vi "Firmware Wizard.vi"() -> ()   [LabVIEW 2011, in "LVH-LINX.lvlib"]
doc: "Wizard for uploading firmware to LINX devices."
uses:
  vi.lib/LabVIEW Hacker/LINX/LVH-LINX.lvlib
  vi.lib/LabVIEW Hacker/LINX/Private/Type Defs/Device Family.ctl
  vi.lib/LabVIEW Hacker/LINX/Private/Type Defs/Devices/Device Type.ctl
  vi.lib/LabVIEW Hacker/LINX/Private/Device/Type Defs/Wifi Config.ctl
  vi.lib/LabVIEW Hacker/LINX/Private/Type Defs/WIFI Security Type.ctl
  vi.lib/LabVIEW Hacker/LINX/Private/Type Defs/Deploy Firmware State.ctl
  vi.lib/LabVIEW Hacker/LINX/Private/Type Defs/All Firmware Data FGV States.ctl
  vi.lib/LabVIEW Hacker/LINX/Private/Device/Type Defs/Firmware Interface.ctl
  vi.lib/LabVIEW Hacker/LINX/Private/Device/Type Defs/TCP Config.ctl
  <vilib>/LabVIEW Hacker/LVH-Toolbox/Common/LVH-Common.lvlib
  vi.lib/LabVIEW Hacker/LINX/Private/Device/Device.lvlib
panel:
  out "Error Out":errorcluster
  out "Log Path":path
  in  "Device Family Enum":T1 items=["National Instruments", "Digilent", "Arduino"]
  in  "Error In":errorcluster
  out "Tab Control":T2(tab)=enum."Device"
  in  "Firmware Available?":string
  in  "Settings Button":bool
  out "Device Image":picture
  in  "Device Help":bool
  in  "Device Type":T3 items=["Arduino Leonardo", "Arduino Mega2560", "Arduino Nano", "Arduino Pro Micro", "Arduino Uno"]
  in  "Device Family":T1 items=["Arduino", "Digilent", "PJRC"]
  in  "Device Cancel":bool
  in  "Device Next":bool
  in  "Firmware Program Interface":u16(ring) items=["Serial / USB"]
  in  "Config Message":string
  in  "Int Help":bool
  in  "Int Previous":bool
  in  "Int Cancel":bool
  in  "Int Next":bool
  out "Interface Config":enum32{"N/A", "Serial / USB", "USB", "TCP"}(tab)=enum."Serial / USB"
  in  "Upload COM Port":refnum<visa-resource-name>="ASRL1::INSTR"
  out "Firmware Configuration":enum32{"Serial", "Ethernet", "WIFI"}(tab)=enum."WIFI"
  in  "Port":u16=927
  in  "IP Address":string="192.168.1.27"
  in  "Wifi Configuration":T4
  in  "Firmware Description":string
  in  "FWV Help":bool
  in  "FWV Cancel":bool
  in  "FWV Next":bool
  in  "FWV Previous":bool
  in  "Firmware Version":u16(ring) items=["LINX - Serial / USB", "LINX - Serial / USB (Debug)"]
  out "Deploy Progress Note":string
  in  "Deploy  Progress Bar":u8(slide) scale=0.0..100.0
  in  "View Log":bool
  in  "LINX Forum Link":string="www.labviewhacker.com/forums/linx"
  in  "LINX Landing Page Link":string="www.labviewhacker.com/linx"
  in  "Summary Launch Example":bool
  in  "Summary Text":string
  in  "Summary Next":bool
  in  "Summary Help":bool
  # "Ethernet Settings"
  # "WIFI Settings"
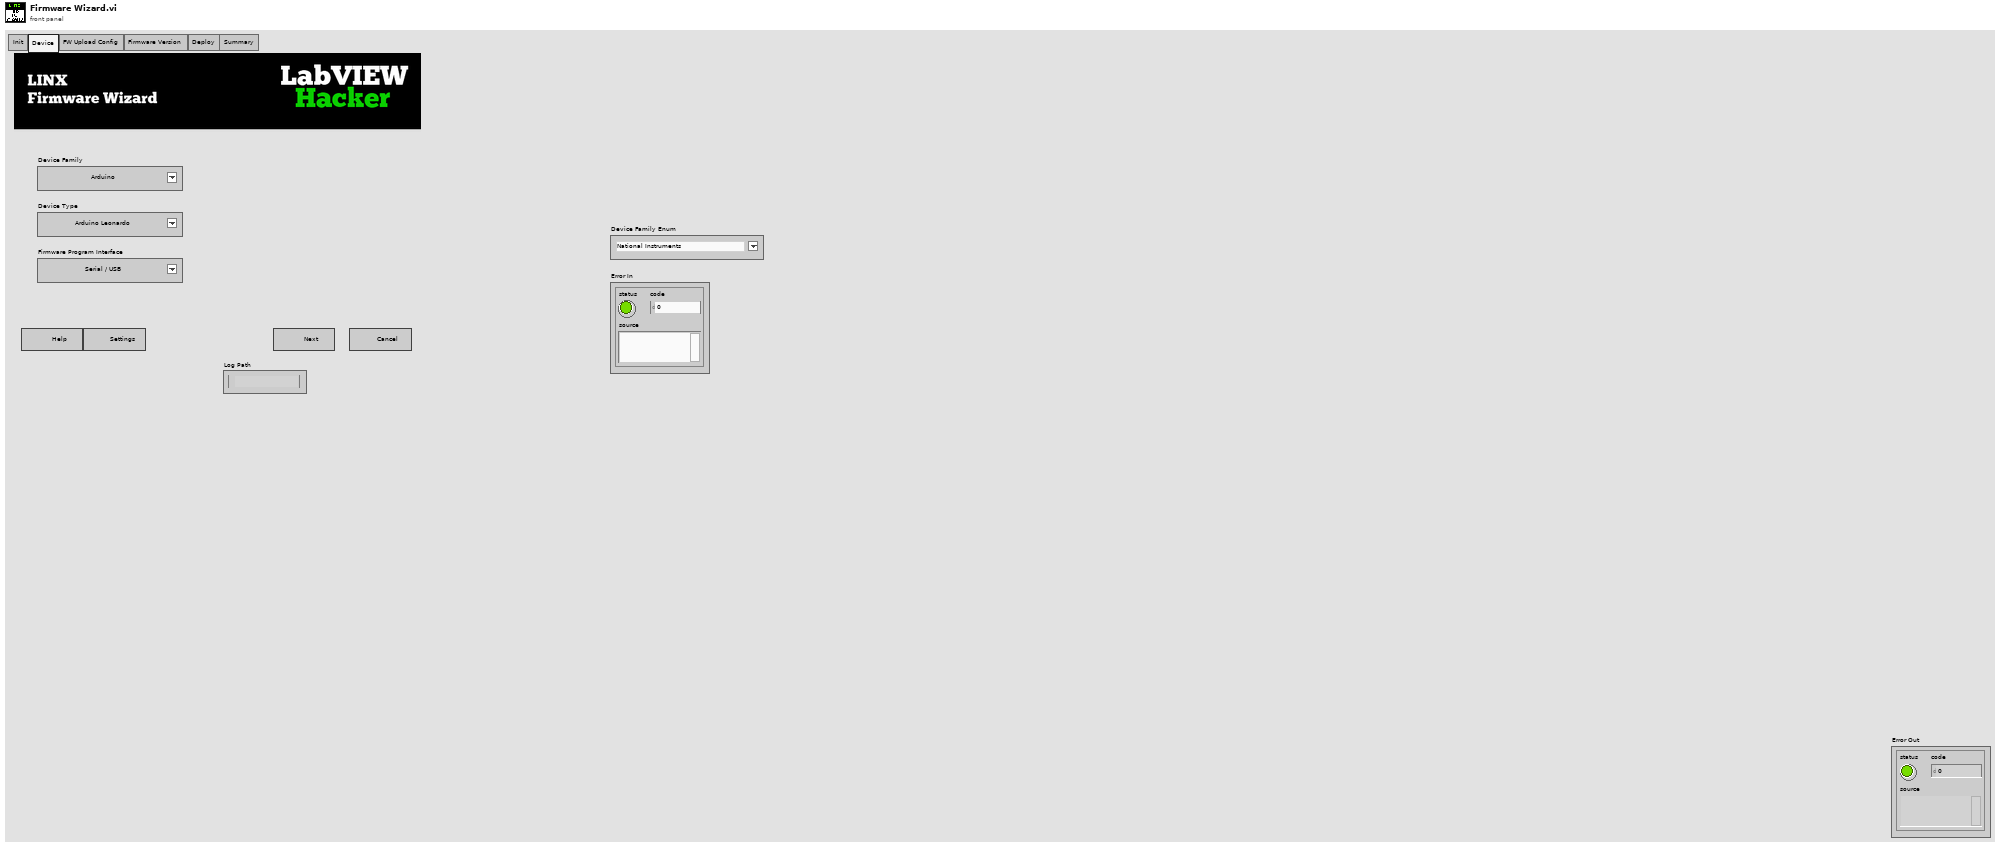
[diagram p1: front panel]
types:
  T1 = typedef "LVH-LINX.lvlib/Device Family.ctl" = u16
  T2 = enum32{"Init", "Device", "FW Upload Config", "Firmware Version", "Deploy", "Summary"}
  T3 = typedef "LVH-LINX.lvlib/Device Type.ctl" = u16
  T4 = typedef "LVH-LINX.lvlib/Device.lvlib/Wifi Config.ctl" = cluster{"SSID":string, "IP Address":string, "Port":u16, "WIFI Security Type":T5, "Password":string}
  T5 = typedef "LVH-LINX.lvlib/WIFI Security Type.ctl" = enum8{"None", "WPA2 Password", "WPA2 Key", "WEP40", "WEP104"}
  T6 = typedef "LVH-LINX.lvlib/Deploy Firmware State.ctl" = enum32{"Init", "Device", "FW Upload Config", "Firmware Version", "Deploy", "Summary"}
  T7 = typedef "LVH-LINX.lvlib/All Firmware Data FGV States.ctl" = enum16{"Set", "Get"}
  T8 = enum8{"Enabled", "Disabled", "Disabled and Grayed Out"}
  T9 = typedef "LVH-LINX.lvlib/Firmware Interface.ctl" = enum32{"Serial ", "Ethernet", "WIFI"}
  T10 = typedef "LVH-LINX.lvlib/Device.lvlib/TCP Config.ctl" = cluster{"IP Address":string, "Port":u16}
  T11 = typedef "LVH-LINX.lvlib/Device Firmware.ctl" = cluster{"Firmware Name":string, "Firmware Path":path, "Description":string, "LINX Interface":string, "Flash Util Working Dir":path, "Flash Util Name":string, "Flash Util Args":string, "Flash Timeout (ms)":i32}
  T12 = enum16{"Left Button", "Center Button", "Right Button", "Window Close"}
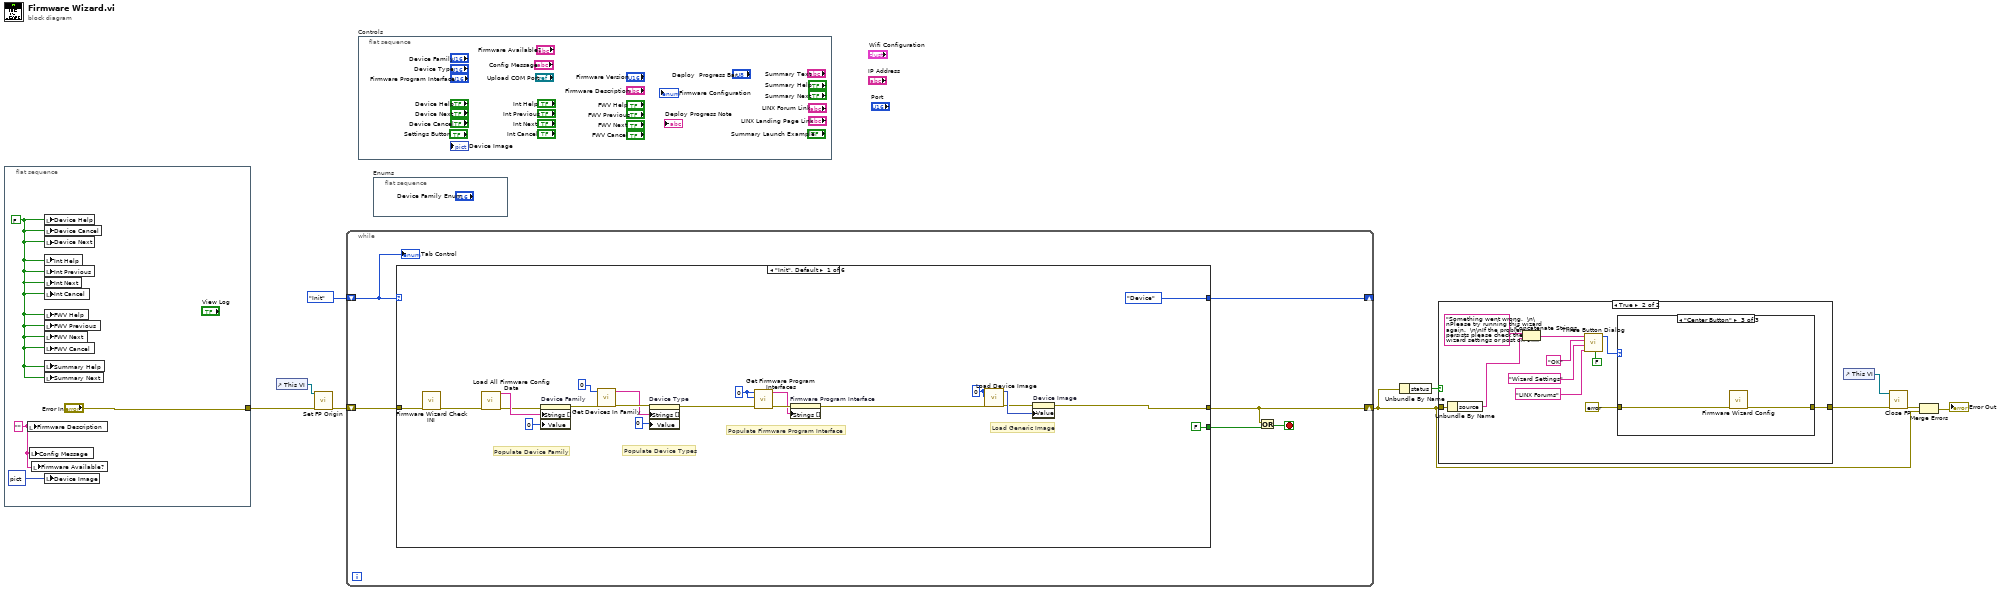
[diagram p0: block diagram]
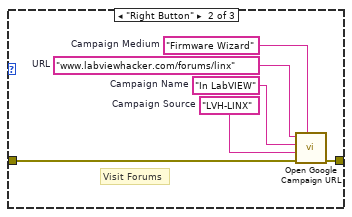
[diagram p4: hidden frame]
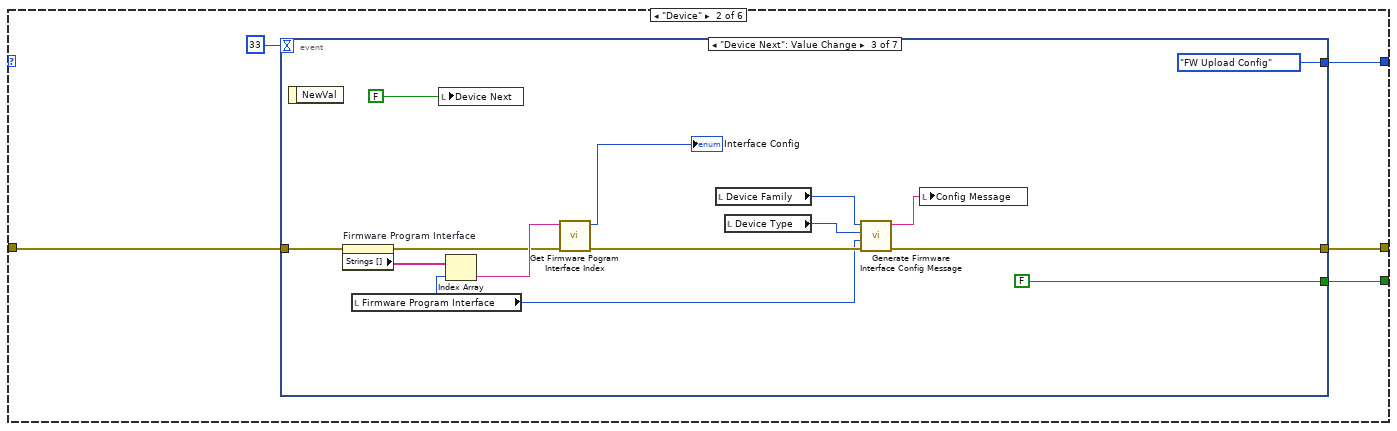
[diagram p5: hidden frame]
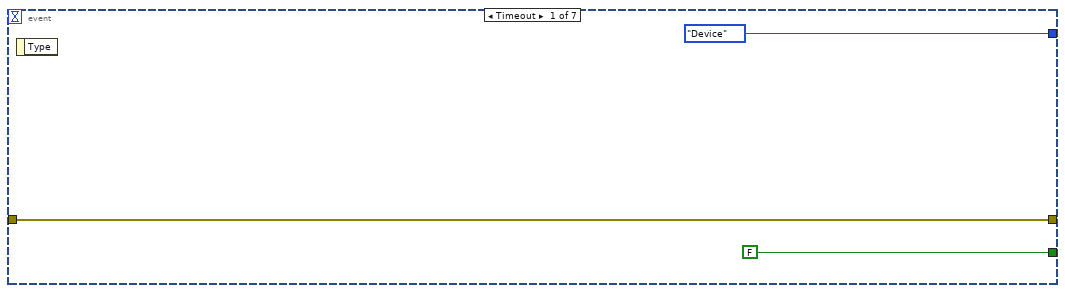
[diagram p6: hidden frame]
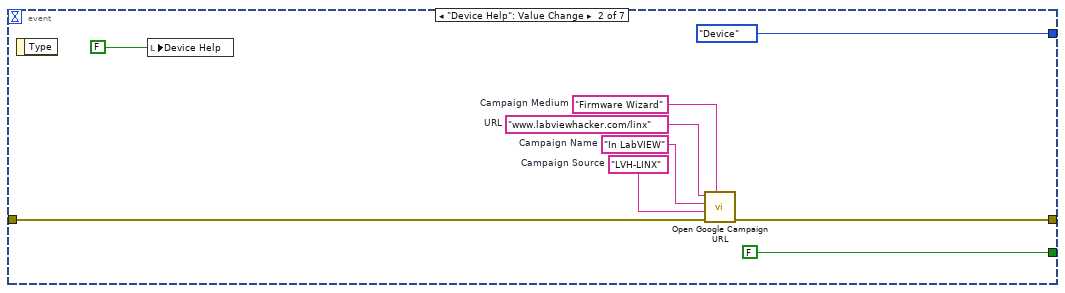
[diagram p7: hidden frame]
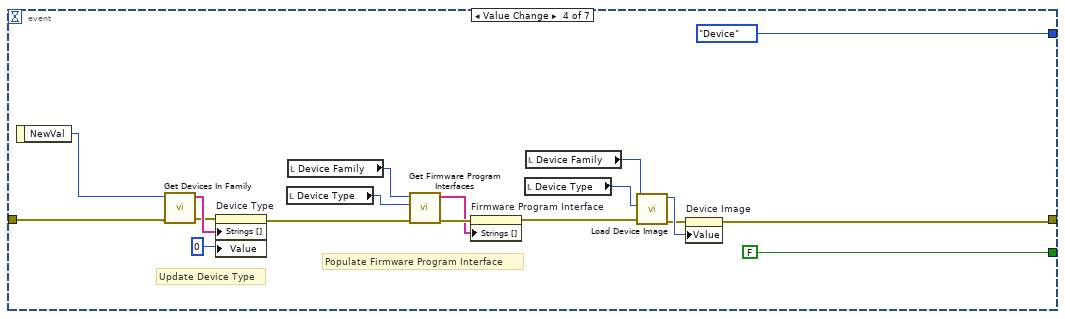
[diagram p8: hidden frame]
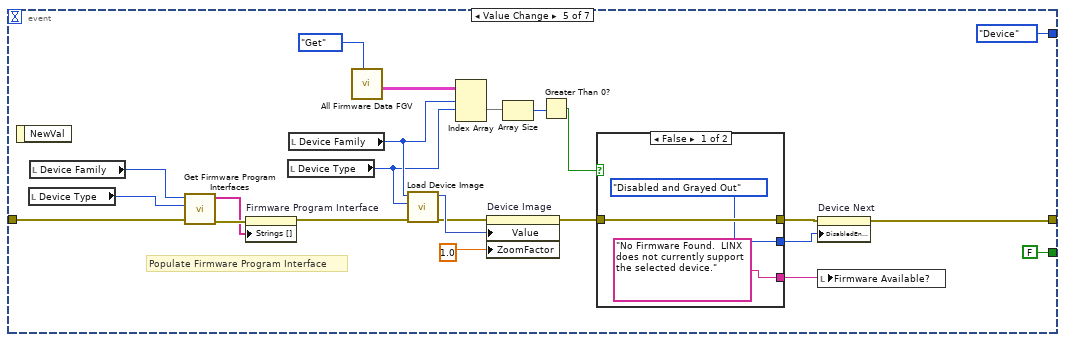
[diagram p9: hidden frame]
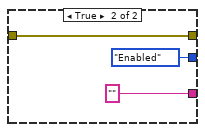
[diagram p10: hidden frame]
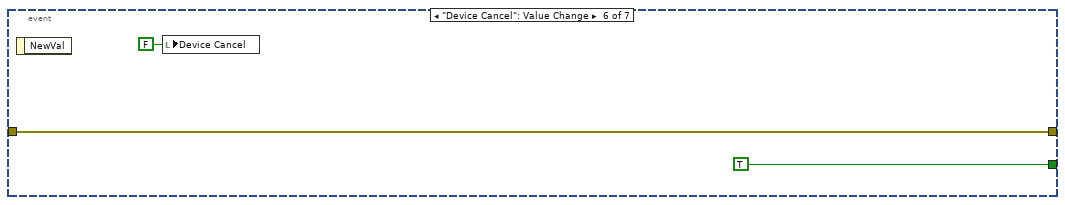
[diagram p11: hidden frame]
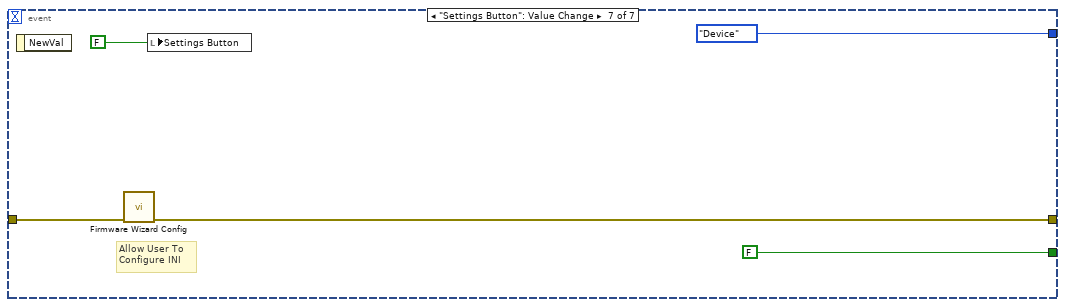
[diagram p12: hidden frame]
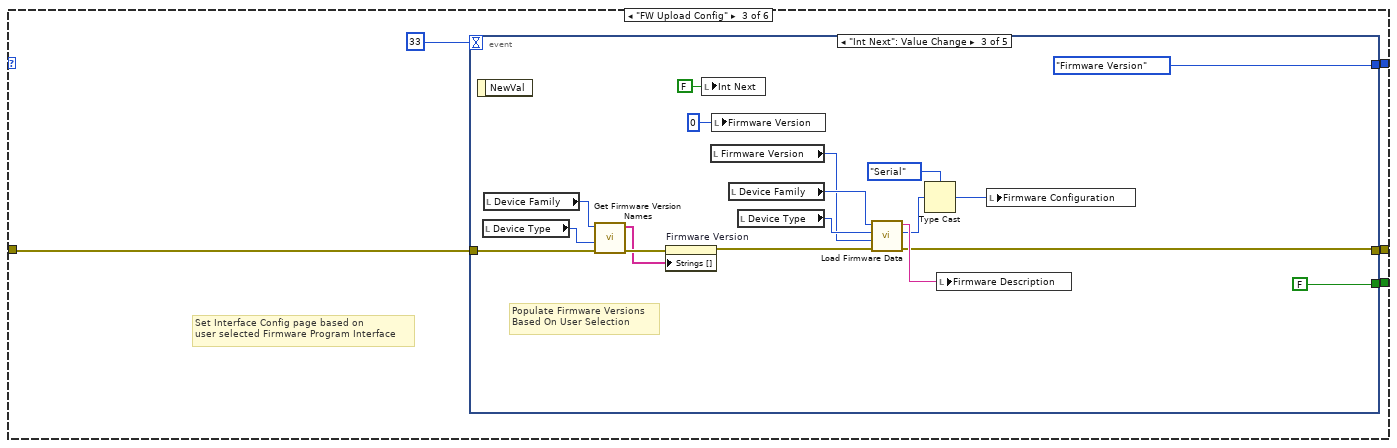
[diagram p13: hidden frame]
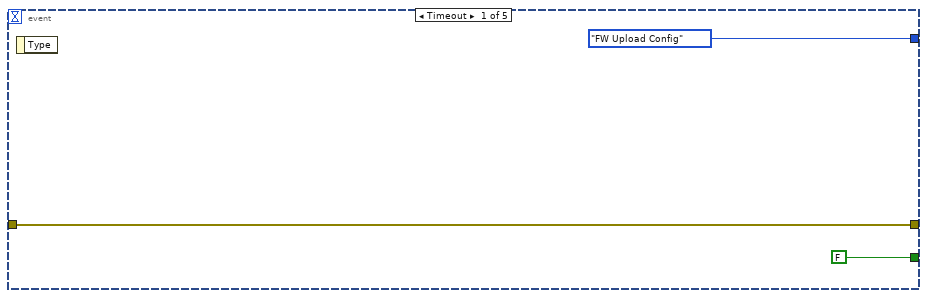
[diagram p14: hidden frame]
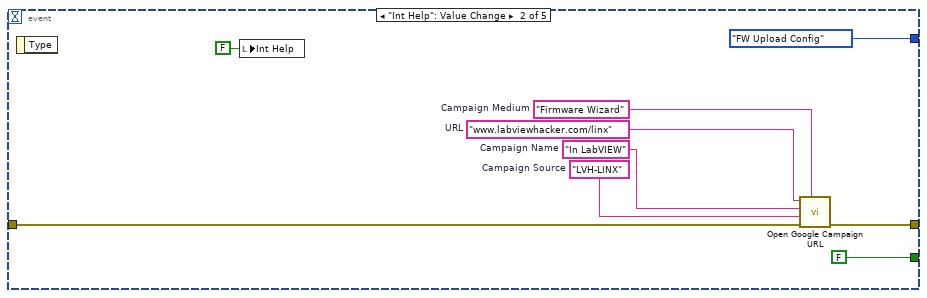
[diagram p15: hidden frame]
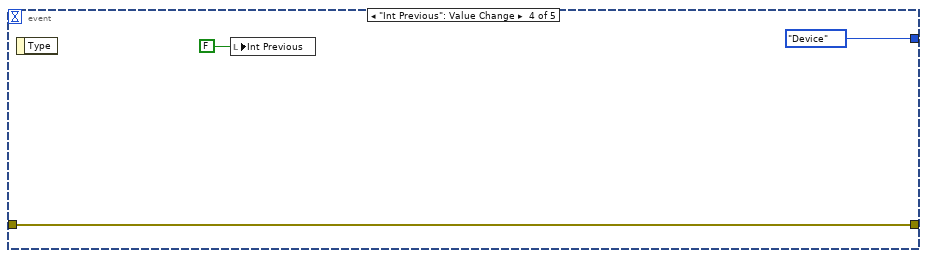
[diagram p16: hidden frame]
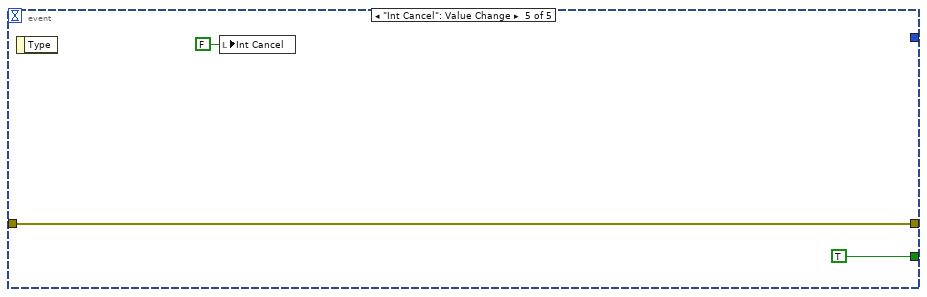
[diagram p17: hidden frame]
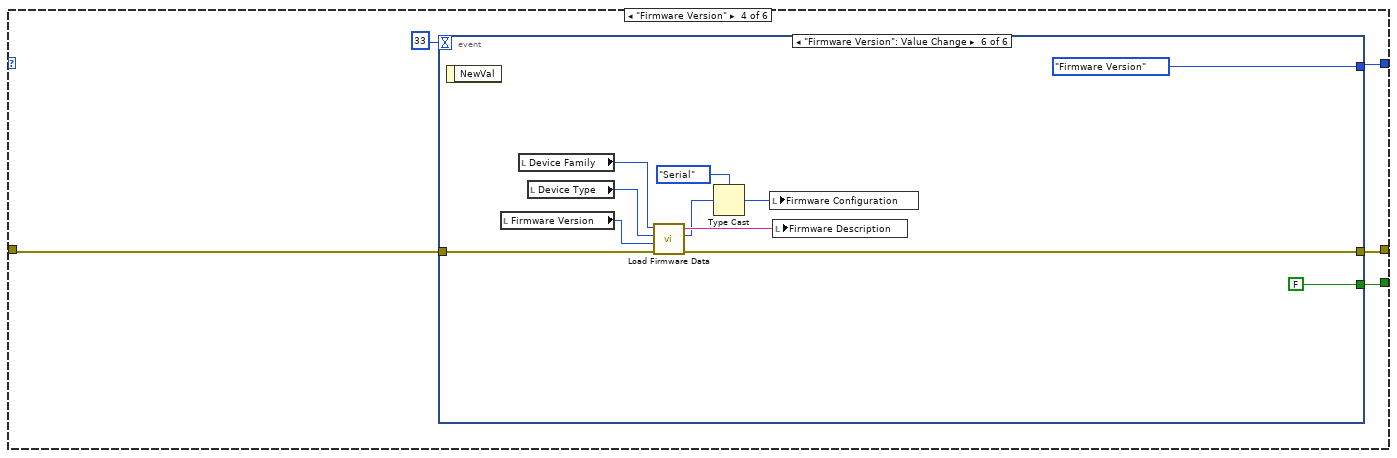
[diagram p18: hidden frame]
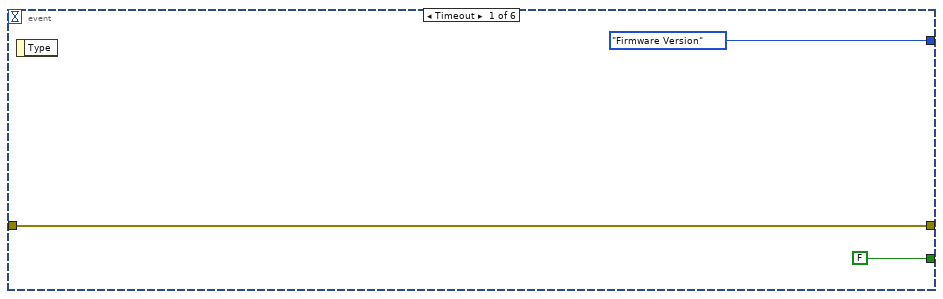
[diagram p19: hidden frame]
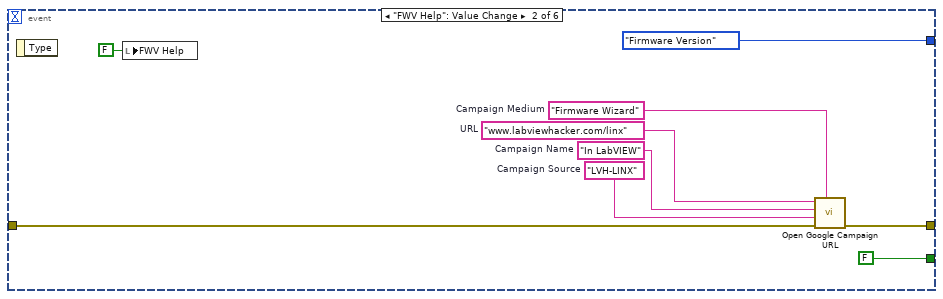
[diagram p20: hidden frame]
diagram:
  n1 = flat-sequence {
    tunnel: ["Error In"] -> w8
    frame #0 {
      w12 = "" ("Firmware Description")
      w14 = FALSE ("Cancel")
      n2 = local write "Firmware Description"(w12) -> ()
      n3 = local write "Config Message"(w12) -> ()
      n4 = local write "Firmware Available?"(w12) -> ()
      n5 = local write "Device Help"(w14) -> ()
      n6 = local write "Device Cancel"(w14) -> ()
      n7 = local write "Device Next"(w14) -> ()
      n8 = local write "Int Help"(w14) -> ()
      n9 = local write "Int Previous"(w14) -> ()
      n10 = local write "Int Next"(w14) -> ()
      n11 = local write "Int Cancel"(w14) -> ()
      n12 = local write "FWV Help"(w14) -> ()
      n13 = local write "FWV Previous"(w14) -> ()
      n14 = local write "FWV Next"(w14) -> ()
      n15 = local write "FWV Cancel"(w14) -> ()
      n16 = local write "Summary Help"(w14) -> ()
      n17 = local write "Summary Next"(w14) -> ()
      n18 = local write "Device Image"(picture data[5B] ("2D Picture")) -> ()
    }
  }
  n19 = control-ref of="This VI"() -> (w9:refnum<vi>)
  n20 = call <vilib>:"Set FP Origin.vi"("Error In"=w8, "VI Ref"=w9) -> ("Error Out"=w7:errorcluster)  [unwired: 9 in]
  n21 = while {
    shift-right: [w18] -> _
    shift-left: Deploy_Firmware_State."Init" ("Deploy Firmware State") -> [w20]
    shift-right: [w17] -> w2
    shift-left: w7 -> [w19]
    stop <- w16 stop-if-true
    n22 = case shown="\"Init\", Default" w20 {
      tunnel: [w31 w45 w131 w173 w209 w250] -> w17
      tunnel: w19 -> [w23 w44 w128 w172 w213 w246]
      tunnel: [Deploy_Firmware_State."Device" ("Deploy Firmware State") w43 w132 w170 Deploy_Firmware_State."Summary" ("Deploy Firmware State") w248] -> w18
      tunnel: [FALSE w42 w129 w169 FALSE w247] -> w15
      frame "Init", Default {
        w24 = 0 ("Device Family Index")
        w35 = 0 ("Device Family")
        # "Load Generic Image"
        # "Populate Firmware Program Interface"
        # "Populate Device Types"
        # "Populate Device Family"
        n23 = call "Firmware Wizard Check INI.vi"("Error In"=w23) -> ("Error Out"=w22:errorcluster)  [unwired: 10 in]
        n24 = call "Load All Firmware Config Data.vi"("Error In"=w22) -> ("Error Out"=w25:errorcluster, "Families"=w26:string[])  [unwired: 7 in, 2 out]
        n25 = property on="Device Family" class="Ring (strict)"(error in=w25, "Strings []"=w26, "Value"=u16 0 ("Device Family")) -> (error out=w30:errorcluster)  [unwired: 1 in, 1 out]
        n26 = call "Get Devices In Family.vi"("Error In"=w30, "Family Index"=0 ("Device Family")) -> ("Error Out"=w29:errorcluster, "Devices"=w28:string[])  [unwired: 8 in]
        n27 = property on="Device Type" class="Ring (strict)"(error in=w29, "Strings []"=w28, "Value"=u16 0 ("Device Family")) -> (error out=w36:errorcluster)  [unwired: 1 in, 1 out]
        n28 = call "Get Firmware Program Interfaces.vi"("Error In"=w36, "Device Index"=w35, "Family Index"=w35) -> ("Error Out"=w38:errorcluster, "Firmware Program Interfaces"=w37:string[])  [unwired: 7 in]
        n29 = property on="Firmware Program Interface" class="Ring (strict)"(error in=w38, "Strings []"=w37) -> (error out=w21:errorcluster)  [unwired: 1 in, 1 out]
        n30 = call "Load Device Image.vi"("Error In"=w21, "Device Index"=w24, "Device Family Index"=w24) -> ("Error Out"=w32:errorcluster, "Device Image"=w33:picture)  [unwired: 6 in, 1 out]
        n31 = property on="Device Image" class="Pict"(error in=w32, "Value"=w33) -> (error out=w31:errorcluster)  [unwired: 1 in, 1 out]
      }
      frame "Device" {
        n32 = event shown="[2] \"Device Next\": Value Change" {
          selector: _ -> [_ _ _ _ _ _ _]
          dyn-events: _ -> [_ _ _ _ _ _ _]
          timeout: 33 -> [_ _ _ _ _ _ _]
          tunnel: [w49 w52 w69 w78 w100 w121 w124] -> w45
          tunnel: w44 -> [w49 w51 w65 w76 w113 w121 w125]
          tunnel: [Deploy_Firmware_State."Device" ("Deploy Firmware State") Deploy_Firmware_State."Device" ("Deploy Firmware State") Deploy_Firmware_State."FW Upload Config" ("Deploy Firmware State") Deploy_Firmware_State."Device" ("Deploy Firmware State") Deploy_Firmware_State."Device" ("Deploy Firmware State") _ Deploy_Firmware_State."Device" ("Deploy Firmware State")] -> w43
          tunnel: [FALSE FALSE FALSE FALSE FALSE TRUE FALSE] -> w42
          event Timeout {
            n33 = event-data() -> ()  [unwired: 1 in, 1 out]
          }
          event "Device Help": Value Change {
            w50 = "LVH-LINX"  # Campaign Source
            w53 = "In LabVIEW"  # Campaign Name
            w54 = "Firmware Wizard"  # Campaign Medium
            w55 = "www.labviewhacker.com/linx"  # URL
            n34 = event-data() -> ()  [unwired: 1 in, 1 out]
            n35 = local write "Device Help"(FALSE ("Device Help")) -> ()
            n36 = call <vilib>:"Open Google Campaign URL.vi"("Campaign Medium"=w54, "Error In"=w51, "Campaign Source"=w50, "Campaign Name"=w53, "URL"=w55) -> ("Error Out"=w52:errorcluster)  [unwired: 5 in, 1 out]
          }
          event "Device Next": Value Change {
            n37 = event-data() -> ()  [unwired: 1 in, 1 out]
            n38 = property on="Firmware Program Interface" class="Ring (strict)"(error in=w65) -> (error out=w66:errorcluster, "Strings []"=w68:string[])  [unwired: 1 in, 1 out]
            n39 = local read "Firmware Program Interface"() -> (w60:u16)
            n40 = local write "Device Next"(FALSE ("Next")) -> ()
            n41 = Index Array(array=w68, index=w60) -> (element=w67:string)
            n42 = call "Get Firmware Pogram Interface Index.vi"("Error In"=w66, "Firmware Program Interface"=w67) -> ("Error Out"=w64:errorcluster, "Interface Index"=→"Interface Config":i32)  [unwired: 8 in]
            n43 = local read "Device Family"() -> (w62:T1)
            n44 = local read "Device Type"() -> (w61:T3)
            n45 = call "Generate Firmware Interface Config Message.vi"("Error In"=w64, "Firmware Program Interface Index"=w60, "Device Index"=w61, "Family Index"=w62) -> ("Error Out"=w69:errorcluster, "Config Message"=w70:string)  [unwired: 6 in]
            n46 = local write "Config Message"(w70) -> ()
          }
          event Value Change {
            # "Populate Firmware Program Interface"
            # "Update Device Type"
            n47 = event-data() -> ("NewVal"=w75:T1)  [unwired: 1 in]
            n48 = call "Get Devices In Family.vi"("Error In"=w76, "Family Index"=w75) -> ("Error Out"=w73:errorcluster, "Devices"=w74:string[])  [unwired: 8 in]
            n49 = property on="Device Type" class="Ring (strict)"(error in=w73, "Strings []"=w74, "Value"=u16 0 ("Device Family")) -> (error out=w85:errorcluster)  [unwired: 1 in, 1 out]
            n50 = local read "Device Type"() -> (w86:T3)
            n51 = local read "Device Family"() -> (w77:T1)
            n52 = call "Get Firmware Program Interfaces.vi"("Error In"=w85, "Device Index"=w86, "Family Index"=w77) -> ("Error Out"=w88:errorcluster, "Firmware Program Interfaces"=w87:string[])  [unwired: 7 in]
            n53 = property on="Firmware Program Interface" class="Ring (strict)"(error in=w88, "Strings []"=w87) -> (error out=w79:errorcluster)  [unwired: 1 in, 1 out]
            n54 = local read "Device Type"() -> (w83:T3)
            n55 = local read "Device Family"() -> (w82:T1)
            n56 = call "Load Device Image.vi"("Error In"=w79, "Device Index"=w83, "Device Family Index"=w82) -> ("Error Out"=w80:errorcluster, "Device Image"=w81:picture)  [unwired: 6 in, 1 out]
            n57 = property on="Device Image" class="Pict"(error in=w80, "Value"=w81) -> (error out=w78:errorcluster)  [unwired: 1 in, 1 out]
          }
          event Value Change {
            # "Populate Firmware Program Interface"
            n58 = event-data() -> ()  [unwired: 1 in, 1 out]
            n59 = local read "Device Type"() -> (w109:T3)
            n60 = local read "Device Family"() -> (w108:T1)
            n61 = call "Get Firmware Program Interfaces.vi"("Error In"=w113, "Device Index"=w109, "Family Index"=w108) -> ("Error Out"=w112:errorcluster, "Firmware Program Interfaces"=w111:string[])  [unwired: 7 in]
            n62 = property on="Firmware Program Interface" class="Ring (strict)"(error in=w112, "Strings []"=w111) -> (error out=w106:errorcluster)  [unwired: 1 in, 1 out]
            n63 = local read "Device Type"() -> (w95:T3)
            n64 = local read "Device Family"() -> (w96:T1)
            n65 = call "All Firmware Data FGV.vi"("All Firmware Data FGV States"=All_Firmware_Data_FGV_States."Get") -> ("Firmwares"=w97:T11[][][])  [unwired: 7 in, 3 out]
            n66 = call "Load Device Image.vi"("Error In"=w106, "Device Index"=w95, "Device Family Index"=w96) -> ("Error Out"=w103:errorcluster, "Device Image"=w105:picture)  [unwired: 6 in, 1 out]
            n67 = Index Array(array=w97, index (dim 0)=w96, index (dim 1)=w95) -> (element=w94:T11[])  [unwired: 1 in]
            n68 = property on="Device Image" class="Pict"(error in=w103, "Value"=w105, "ZoomFactor"=sgl 1.0 ("Zoom Factor")) -> (error out=w102:errorcluster)  [unwired: 1 in, 1 out]
            n69 = Array Size(array=w94) -> (size(s)=w93:i32)
            n70 = Greater Than 0?(x=w93) -> (x > 0?=w92:bool)
            n71 = case shown="False" w92 {
              tunnel: [w116 w119] -> w101
              tunnel: w102 -> [w116 w119]
              tunnel: [T8."Disabled and Grayed Out" ("Disabled") T8."Enabled" ("Disabled")] -> w99
              tunnel: ["No Firmware Found.  LINX does not currently support the selected device." ("Firmware Available?") "" ("Firmware Available?")] -> w98
              frame False {
              }
              frame True {
              }
            }
            n72 = property on="Device Next" class="Bool (strict)"(error in=w101, "DisabledEnum"=w99) -> (error out=w100:errorcluster)  [unwired: 1 in, 1 out]
            n73 = local write "Firmware Available?"(w98) -> ()
          }
          event "Device Cancel": Value Change {
            n74 = event-data() -> ()  [unwired: 1 in, 1 out]
            n75 = local write "Device Cancel"(FALSE ("Device Cancel")) -> ()
          }
          event "Settings Button": Value Change {
            # "Allow User To \nConfigure INI"
            n76 = event-data() -> ()  [unwired: 1 in, 1 out]
            n77 = call "Firmware Wizard Config.vi"("Error In"=w125) -> ("Error Out"=w124:errorcluster)  [unwired: 10 in]
            n78 = local write "Settings Button"(FALSE ("Settings Button")) -> ()
          }
        }
      }
      frame "FW Upload Config" {
        # "Set Interface Config page based on \nuser selected Firmware Program Interface"
        n79 = event shown="[2] \"Int Next\": Value Change" {
          selector: _ -> [_ _ _ _ _]
          dyn-events: _ -> [_ _ _ _ _]
          timeout: 33 -> [_ _ _ _ _]
          tunnel: [Deploy_Firmware_State."FW Upload Config" ("Deploy Firmware State") Deploy_Firmware_State."FW Upload Config" ("Deploy Firmware State") Deploy_Firmware_State."Firmware Version" ("Deploy Firmware State") Deploy_Firmware_State."Device" ("Deploy Firmware State") _] -> w132
          tunnel: [w134 w136 w149 w165 w166] -> w131
          tunnel: w128 -> [w134 w137 w162 w165 w166]
          tunnel: [FALSE FALSE FALSE _ TRUE] -> w129
          event Timeout {
            n80 = event-data() -> ()  [unwired: 1 in, 1 out]
          }
          event "Int Help": Value Change {
            w138 = "LVH-LINX"  # Campaign Source
            w139 = "In LabVIEW"  # Campaign Name
            w140 = "Firmware Wizard"  # Campaign Medium
            w141 = "www.labviewhacker.com/linx"  # URL
            n81 = event-data() -> ()  [unwired: 1 in, 1 out]
            n82 = local write "Int Help"(FALSE ("Int Help")) -> ()
            n83 = call <vilib>:"Open Google Campaign URL.vi"("Campaign Medium"=w140, "Error In"=w137, "Campaign Source"=w138, "Campaign Name"=w139, "URL"=w141) -> ("Error Out"=w136:errorcluster)  [unwired: 5 in, 1 out]
          }
          event "Int Next": Value Change {
            # "Populate Firmware Versions\nBased On User Selection"
            n84 = event-data() -> ()  [unwired: 1 in, 1 out]
            n85 = local read "Device Type"() -> (w159:T3)
            n86 = local read "Device Family"() -> (w158:T1)
            n87 = call "Get Firmware Version Names.vi"("Error In"=w162, "Device Index"=w159, "Family Index"=w158) -> ("Error Out"=w161:errorcluster, "Firmware Version Names"=w160:string[])  [unwired: 6 in, 1 out]
            n88 = property on="Firmware Version" class="Ring (strict)"(error in=w161, "Strings []"=w160) -> (error out=w153:errorcluster)  [unwired: 1 in, 1 out]
            n89 = local write "Int Next"(FALSE ("Int Next")) -> ()
            n90 = local read "Firmware Version"() -> (w146:u16)
            n91 = local write "Firmware Version"(0) -> ()
            n92 = local read "Device Family"() -> (w148:T1)
            n93 = local read "Device Type"() -> (w147:T3)
            n94 = call "Load Firmware Data.vi"("Error In"=w153, "Firmware Index"=w146, "Device Index"=w147, "Family Index"=w148) -> ("Error Out"=w149:errorcluster, "Firmware Interface"=w145:T9, "Firmware Description"=w154:string)  [unwired: 5 in]
            n95 = Type Cast(type=enum32{"Serial", "Ethernet", "WIFI"}."Serial" ("Firmware Configuration"), x=w145) -> (*(type *) &x=w150:enum32{"Serial", "Ethernet", "WIFI"})
            n96 = local write "Firmware Description"(w154) -> ()
            n97 = local write "Firmware Configuration"(w150) -> ()
          }
          event "Int Previous": Value Change {
            n98 = event-data() -> ()  [unwired: 1 in, 1 out]
            n99 = local write "Int Previous"(FALSE ("Previous")) -> ()
          }
          event "Int Cancel": Value Change {
            n100 = event-data() -> ()  [unwired: 1 in, 1 out]
            n101 = local write "Int Cancel"(FALSE ("Int Cancel")) -> ()
          }
        }
      }
      frame "Firmware Version" {
        n102 = event shown="[5] \"Firmware Version\": Value Change" {
          selector: _ -> [_ _ _ _ _ _]
          dyn-events: _ -> [_ _ _ _ _ _]
          timeout: 33 -> [_ _ _ _ _ _]
          tunnel: [w176 w178 w188 w192 w196 w205] -> w173
          tunnel: w172 -> [w176 w177 w188 w192 w196 w206]
          tunnel: [Deploy_Firmware_State."Firmware Version" ("Deploy Firmware State") Deploy_Firmware_State."Firmware Version" ("Deploy Firmware State") Deploy_Firmware_State."FW Upload Config" ("Deploy Firmware State") Deploy_Firmware_State."Deploy" ("Deploy Firmware State") Deploy_Firmware_State."Init" ("Deploy Firmware State") Deploy_Firmware_State."Firmware Version" ("Deploy Firmware State")] -> w170
          tunnel: [FALSE FALSE FALSE FALSE TRUE FALSE] -> w169
          event Timeout {
            n103 = event-data() -> ()  [unwired: 1 in, 1 out]
          }
          event "FWV Help": Value Change {
            w179 = "LVH-LINX"  # Campaign Source
            w180 = "In LabVIEW"  # Campaign Name
            w181 = "Firmware Wizard"  # Campaign Medium
            w182 = "www.labviewhacker.com/linx"  # URL
            n104 = event-data() -> ()  [unwired: 1 in, 1 out]
            n105 = local write "FWV Help"(FALSE ("FWV Help")) -> ()
            n106 = call <vilib>:"Open Google Campaign URL.vi"("Campaign Medium"=w181, "Error In"=w177, "Campaign Source"=w179, "Campaign Name"=w180, "URL"=w182) -> ("Error Out"=w178:errorcluster)  [unwired: 5 in, 1 out]
          }
          event "FWV Previous": Value Change {
            n107 = event-data() -> ()  [unwired: 1 in, 1 out]
            n108 = local write "FWV Previous"(FALSE ("FWV Previous")) -> ()
          }
          event "FWV Next": Value Change {
            n109 = event-data() -> ()  [unwired: 1 in, 1 out]
            n110 = local write "FWV Next"(FALSE ("FWV Previous")) -> ()
          }
          event "FWV Cancel": Value Change {
            n111 = event-data() -> ()  [unwired: 1 in, 1 out]
            n112 = local write "FWV Cancel"(FALSE ("FWV Previous")) -> ()
          }
          event "Firmware Version": Value Change {
            n113 = event-data() -> ()  [unwired: 1 in, 1 out]
            n114 = local read "Firmware Version"() -> (w198:u16)
            n115 = local read "Device Family"() -> (w200:T1)
            n116 = local read "Device Type"() -> (w199:T3)
            n117 = call "Load Firmware Data.vi"("Error In"=w206, "Firmware Index"=w198, "Device Index"=w199, "Family Index"=w200) -> ("Error Out"=w205:errorcluster, "Firmware Interface"=w202:T9, "Firmware Description"=w204:string)  [unwired: 5 in]
            n118 = Type Cast(type=enum32{"Serial", "Ethernet", "WIFI"}."Serial" ("Firmware Configuration"), x=w202) -> (*(type *) &x=w201:enum32{"Serial", "Ethernet", "WIFI"})
            n119 = local write "Firmware Configuration"(w201) -> ()
            n120 = local write "Firmware Description"(w204) -> ()
          }
        }
      }
      frame "Deploy" {
        n121 = flat-sequence {
          tunnel: w213 -> [w218]
          tunnel: [w218] -> w212
          tunnel: [w224] -> w215
          tunnel: [w223] -> w214
          tunnel: w212 -> [w222]
          tunnel: w215 -> [w229]
          tunnel: w214 -> [w228]
          tunnel: [w229] -> w211
          tunnel: [w228] -> w210
          tunnel: w211 -> [w238]
          tunnel: w210 -> [w237]
          tunnel: [w232] -> w209
          frame #0 {
            n122 = local write "Deploy Progress Note"("Uploading Device Firmware" ("Deploy Progress Note")) -> ()
          }
          frame #1 {
            n123 = local read "Firmware Version"() -> (w221:u16)
            n124 = local read "Upload COM Port"() -> (w223:refnum<visa-resource-name>)
            n125 = local read "Device Family"() -> (w226:T1)
            n126 = local read "Device Type"() -> (w225:T3)
            n127 = control-ref of="Deploy  Progress Bar"() -> (w227:refnum<vi>)
            n128 = call "Upload Firmware.vi"("Progress Bar"=w227, "COM Port"=w223, "Error In"=w222, "Firmware Index"=w221, "Device Index"=w225, "Family Index"=w226) -> ("Error Out"=w224:errorcluster, "Log Path"=→"Log Path":path)  [unwired: 4 in]
          }
          frame #2 {
            n129 = local write "Deploy Progress Note"("Configuring Device Settings" ("Deploy Progress Note")) -> ()
          }
          frame #3 {
            n130 = local read "Firmware Configuration"() -> (w234:enum32{"Serial", "Ethernet", "WIFI"})
            n131 = local read "IP Address"() -> (w241:string)
            n132 = local read "Port"() -> (w240:u16)
            n133 = local read "Wifi Configuration"() -> (w231:T4)
            n134 = Bundle By Name(cluster=T10 {"IP Address"="", "Port"=0} ("TCP Configuration"), "IP Address"=w241, "Port"=w240) -> (w236:T10)
            n135 = Type Cast(type=Firmware_Interface."Serial " ("Firmware Interface"), x=w234) -> (*(type *) &x=w235:T9)
            n136 = call "Configure LINX Device.vi"("Wifi Configuration"=w231, "TCP Configuration"=w236, "Error In"=w238, "Firmware Interface"=w235, "COM Port"=w237) -> ("Error Out"=w232:errorcluster)  [unwired: 6 in]
          }
        }
      }
      frame "Summary" {
        n137 = local read "Device Family"() -> (w244:T1)
        n138 = local read "Device Type"() -> (w243:T3)
        n139 = call "Generate Firmware Wizard Summary Message.vi"("Error In"=w246, "Device ID"=w243, "Device Family"=w244) -> ("Error Out"=w245:errorcluster, "Summary"=w242:string)  [unwired: 7 in]
        n140 = local write "Summary Text"(w242) -> ()
        n141 = event shown="[4] \"View Log\": Value Change" {
          selector: _ -> [_ _ _ _ _ _ _]
          dyn-events: _ -> [_ _ _ _ _ _ _]
          timeout: 33 -> [_ _ _ _ _ _ _]
          tunnel: [w253 w260 w267 w275 w277 w291 w314] -> w250
          tunnel: w245 -> [w253 w259 w266 w274 w276 w300 w314]
          tunnel: [Deploy_Firmware_State."Summary" ("Deploy Firmware State") Deploy_Firmware_State."Summary" ("Deploy Firmware State") Deploy_Firmware_State."Summary" ("Deploy Firmware State") Deploy_Firmware_State."Summary" ("Deploy Firmware State") Deploy_Firmware_State."Summary" ("Deploy Firmware State") Deploy_Firmware_State."Summary" ("Deploy Firmware State") Deploy_Firmware_State."Init" ("Deploy Firmware State")] -> w248
          tunnel: [FALSE _ _ _ _ TRUE TRUE] -> w247
          event Timeout {
            n142 = event-data() -> ()  [unwired: 1 in, 1 out]
          }
          event "LINX Forum Link": Mouse Down {
            w255 = "LVH-LINX"  # Campaign Source
            w256 = "In LabVIEW"  # Campaign Name
            w257 = "Firmware Wizard"  # Campaign Medium
            w258 = "www.labviewhacker.com/forums/linx"  # URL
            n143 = event-data() -> ()  [unwired: 1 in, 7 out]
            n144 = call <vilib>:"Open Google Campaign URL.vi"("Campaign Medium"=w257, "Error In"=w259, "Campaign Source"=w255, "Campaign Name"=w256, "URL"=w258) -> ("Error Out"=w260:errorcluster)  [unwired: 5 in, 1 out]
          }
          event "LINX Landing Page Link": Mouse Down {
            w262 = "LVH-LINX"  # Campaign Source
            w263 = "In LabVIEW"  # Campaign Name
            w264 = "Firmware Wizard"  # Campaign Medium
            w265 = "www.labviewhacker.com/linx"  # URL
            n145 = event-data() -> ()  [unwired: 1 in, 7 out]
            n146 = call <vilib>:"Open Google Campaign URL.vi"("Campaign Medium"=w264, "Error In"=w266, "Campaign Source"=w262, "Campaign Name"=w263, "URL"=w265) -> ("Error Out"=w267:errorcluster)  [unwired: 5 in, 1 out]
          }
          event "Summary Help": Value Change {
            w270 = "LVH-LINX"  # Campaign Source
            w271 = "In LabVIEW"  # Campaign Name
            w272 = "Firmware Wizard"  # Campaign Medium
            w273 = "www.labviewhacker.com/linx"  # URL
            n147 = event-data() -> ()  [unwired: 1 in, 1 out]
            n148 = local write "Summary Help"(FALSE ("Summary Help")) -> ()
            n149 = call <vilib>:"Open Google Campaign URL.vi"("Campaign Medium"=w272, "Error In"=w274, "Campaign Source"=w270, "Campaign Name"=w271, "URL"=w273) -> ("Error Out"=w275:errorcluster)  [unwired: 5 in, 1 out]
          }
          event "View Log": Value Change {
            w283 = "\"" ("string")
            # "Open Log File In Default Text Editor"
            n150 = event-data() -> ()  [unwired: 1 in, 5 out]
            n151 = local write "View Log"(FALSE ("Summary Help")) -> ()
            n152 = local read "Log Path"() -> (w278:path)
            n153 = Path To String(path=w278) -> (string=w284:string)
            n154 = Concatenate Strings("cmd /k" ("command line"), w283, w284, w283) -> (w281:string)
            n155 = call <vilib>:"System Exec.vi"("run minimized? (F)"=TRUE, "wait until completion? (T)"=FALSE, "error in (no error)"=w276, "command line"=w281) -> ("error out"=w277:errorcluster)  [unwired: 4 in, 3 out]
          }
          event "Summary Launch Example": Value Change {
            n156 = event-data() -> ()  [unwired: 1 in, 1 out]
            n157 = local read "Firmware Configuration"() -> (w307:enum32{"Serial", "Ethernet", "WIFI"})
            n158 = call <vilib>:"Get Main Path.vi"("Error In"=w300) -> ("Error Out"=w301:errorcluster, "Main Dir"=w303:path)  [unwired: 8 in, 1 out]
            n159 = local write "Summary Launch Example"(FALSE ("Summary Launch Example")) -> ()
            n160 = call <vilib>:"Strip Path To Token.vi"("Error In"=w301, "Token (Regex)"="LabVIEW [0-9]+.?[0-9]?", "Path"=w303) -> ("Error Out"=w299:errorcluster, "Stripped Path"=w304:path)  [unwired: 6 in, 1 out]
            n161 = call <vilib>:"Append Relative Path String.vi"("Error In"=w299, "Relative Path"="\\examples\\LabVIEW Hacker\\LINX", "Base Path"=w304) -> ("Error Out"=w290:errorcluster, "Absolute Path"=w289:path)  [unwired: 7 in]
            n162 = Type Cast(type=Firmware_Interface."Serial " ("Firmware Interface"), x=w307) -> (*(type *) &x=w305:T9)
            n163 = case shown="\"Ethernet\", \"WIFI\"" w305 {
              tunnel: ["LINX - Blink (Simple).vi" ("name or relative path") "LINX - Blink (Simple) (TCP).vi" ("name or relative path")] -> w288
              frame "Serial ", Default {
              }
              frame "Ethernet", "WIFI" {
              }
            }
            n164 = Build Path(base path=w289, name or relative path=w288) -> (appended path=w297:path)
            n165 = Open VI Reference(vi path=w297, error in (no error)=w290) -> (vi reference=w296:refnum<vi>, error out=w295:errorcluster)  [unwired: 4 in]
            n166 = property class="VI"(reference=w296, error in=w295, "Front Panel.Open"=TRUE ("Front Panel Window:Open")) -> (reference out=w292:refnum<vi>, error out=w293:errorcluster)
            n167 = Close Reference(reference=w292, error in (no error)=w293) -> (error out=w291:errorcluster)
          }
          event "Summary Next": Value Change {
            n168 = event-data() -> ()  [unwired: 1 in, 1 out]
            n169 = local write "Summary Next"(FALSE ("FWV Previous")) -> ()
          }
        }
      }
    }
    n170 = Or(x=w17, y=w15) -> (x .or. y?=w16:bool)
    "Tab Control" <- w20
  }
  n171 = flat-sequence "Controls" {
    frame #0 {
    }
  }
  n172 = flat-sequence "Enums" {
    frame #0 {
    }
  }
  n173 = Unbundle By Name(w2) -> ("status"=w6:bool)
  n174 = case shown="True" w6 {
    tunnel: [w316 w326] -> w5
    tunnel: w2 -> [w316 w318]
    frame False {
    }
    frame True {
      n175 = Unbundle By Name(w318) -> ("source"=w317:string)
      n176 = Concatenate Strings("Something went wrong.  \n\nPlease try running this wizard again.  \n\nIf the problem persists please check the wizard settings or post on the LVH LINX Forums at: \n\nwww.labviewhacker.com/forums/linx \n\n", w317) -> (w319:string)
      n177 = call <vilib>:"Three Button Dialog.vi"("Allow user to close window? (TRUE)"=FALSE, "Right Button Text (\"Cancel\")"="LINX Forums" ("F button name (\"Cancel\")"), "Center Button Text (\"No\")"="Wizard Settings" ("F button name (\"Cancel\")"), "Left Button Text (\"Yes\")"="OK" ("Left Button Text (\"Yes\")"), "message"=w319) -> ("Which Button?"=w321:T12)  [unwired: 6 in]
      n178 = case shown="\"Center Button\"" w321 {
        tunnel: errorcluster {"status"=FALSE, "code"=0, "source"=""} ("error constant") -> [w328 w330 w336]
        tunnel: [w328 w329 w335] -> w326
        frame "Left Button", Default {
          # "Nothing To Do Here"
        }
        frame "Right Button" {
          w331 = "LVH-LINX"  # Campaign Source
          w332 = "In LabVIEW"  # Campaign Name
          w333 = "Firmware Wizard"  # Campaign Medium
          w334 = "www.labviewhacker.com/forums/linx"  # URL
          # "Visit Forums"
          n179 = call <vilib>:"Open Google Campaign URL.vi"("Campaign Medium"=w333, "Error In"=w330, "Campaign Source"=w331, "Campaign Name"=w332, "URL"=w334) -> ("Error Out"=w329:errorcluster)  [unwired: 5 in, 1 out]
        }
        frame "Center Button" {
          n180 = call "Firmware Wizard Config.vi"("Error In"=w336) -> ("Error Out"=w335:errorcluster)  [unwired: 10 in]
        }
      }
    }
  }
  n181 = control-ref of="This VI"() -> (w4:refnum<vi>)
  n182 = call <vilib>:"Close FP.vi"("Error In"=w5, "VI Ref"=w4) -> ("Error Out"=w3:errorcluster)  [unwired: 9 in]
  n183 = Merge Errors(w3, w2) -> (→"Error Out":errorcluster)
